vi "G Primitive to PLC Byte Stream.vi"(6 "Byte Length":i32, 8 "error in (no error)":errorcluster, 9 "PLC Type":T1, 10 "Value":variant, 11 "TwinCAT ADS in":refnum<class "TwinCAT ADS.lvclass">) -> (0 "error out":errorcluster, 2 "Byte Stream":u8[](array[numeric]), 3 "TwinCAT ADS out":refnum<class "TwinCAT ADS.lvclass">)   [LabVIEW 2018, in "TwinCAT ADS.lvclass"]
uses:
  TwinCAT ADS.lvclass
  Controls/PLC Type.ctl
  ebfc1059-5ad7-41af-9a32-6ba056cec1e2.vi
  6e01a951-886b-41b5-8cd1-fdd71fd1a533.vi
  09c7a0ef-3209-4624-b801-f77696e71225.vi
  97b8602c-6a72-408e-90bf-08a26de32539.vi
  0fd4fbf3-4a18-432c-8f70-6a5c8fef8454.vi
  afdb5a5e-237c-4be5-828e-15f510cf6cea.vi
  185a6e12-4d7d-4ad7-9936-0525adb2f85e.vi
  88229fb8-b58c-494b-bd2b-fea6e0d0ed1b.vi
  e57df404-389c-41d0-a67c-37c75754ab31.vi
  d0ee652c-9b86-46ed-9065-57d03aa8de3e.vi
  886bf0b9-f01c-4a44-b2e2-abccc7b97bfa.vi
  35f71df7-fc14-4c4d-983c-cf72c138dc9e.vi
  2d2bc992-a9ff-4dd8-b8fe-74c21cb85899.vi
  100e4a11-5e4a-45b7-be98-adc9eaebd48d.vi
  132946d9-68c7-4ade-a66d-dc369520c644.vi
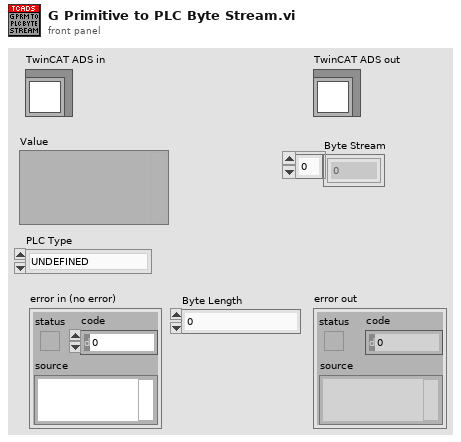
[diagram p1: front panel]
types:
  T1 = typedef "TwinCAT ADS.lvclass/PLC Type.ctl" = enum16{"UNDEFINED", "INT", "DINT", "REAL", "LREAL", "SINT", "BYTE", "UINT", "UDINT", "LINT", "ULINT", "STRING", "WSTRING", "BOOL", "TIME", "LTIME", "DATE", "DT", "TOD", "ARRAY", "JAGGED ARRAY", "STRUCT", "FUNCTION BLOCK", "UNION", "POINTER", "USER DEFINED"}
  T2 = typedef "LVDateTimeRec.ctl" = cluster{"fractional second":dbl, "second":i32, "minute":i32, "hour":i32, "day of month":i32, "month":i32, "year":i32, "day of week":i32, "day of year":i32, "DST":i32}
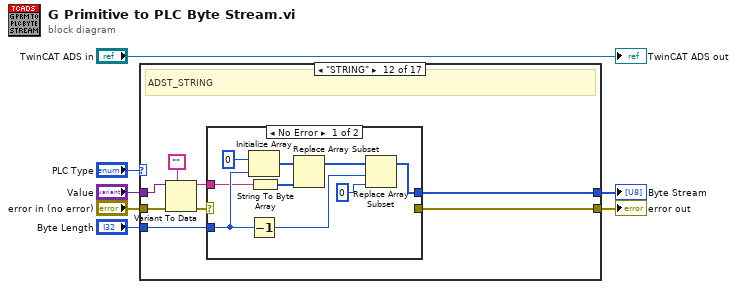
[diagram p0: block diagram]
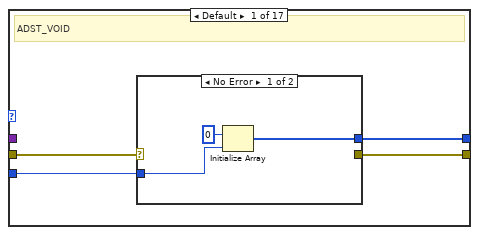
[diagram p2: hidden frame]
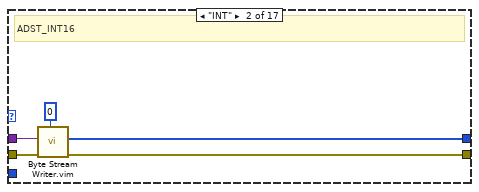
[diagram p4: hidden frame]
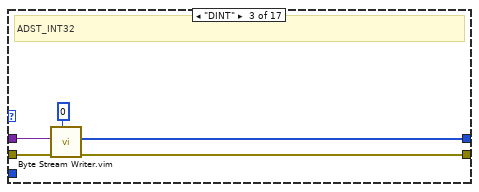
[diagram p5: hidden frame]
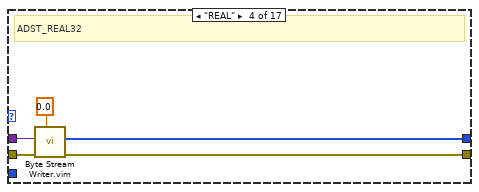
[diagram p6: hidden frame]
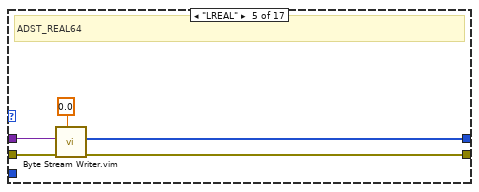
[diagram p7: hidden frame]
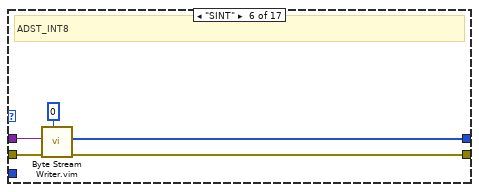
[diagram p8: hidden frame]
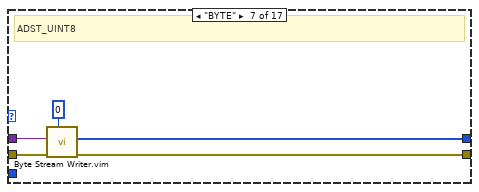
[diagram p9: hidden frame]
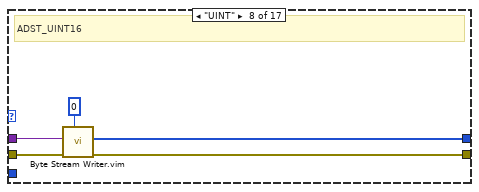
[diagram p10: hidden frame]
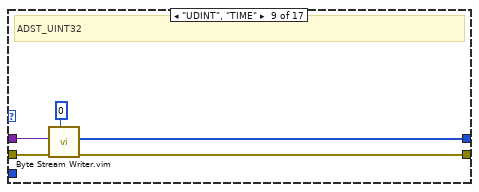
[diagram p11: hidden frame]
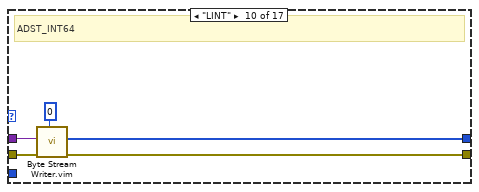
[diagram p12: hidden frame]
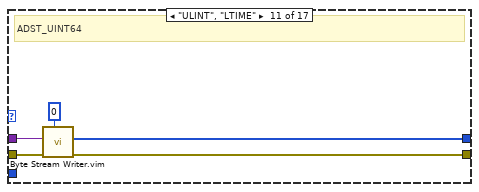
[diagram p13: hidden frame]
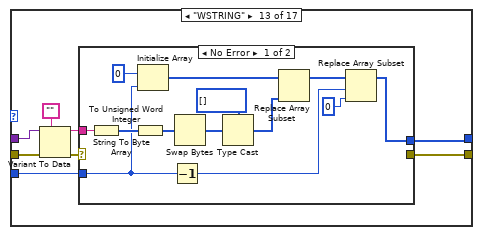
[diagram p15: hidden frame]
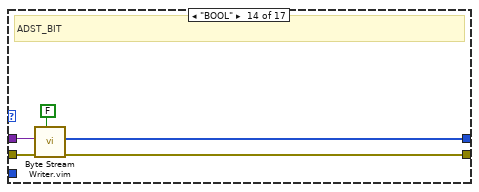
[diagram p17: hidden frame]
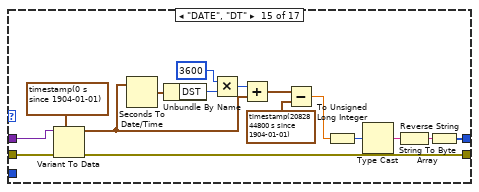
[diagram p18: hidden frame]
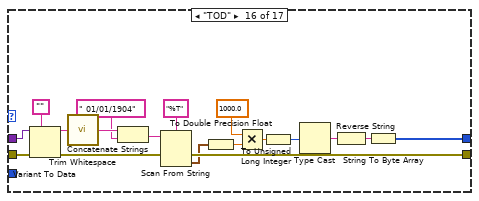
[diagram p19: hidden frame]
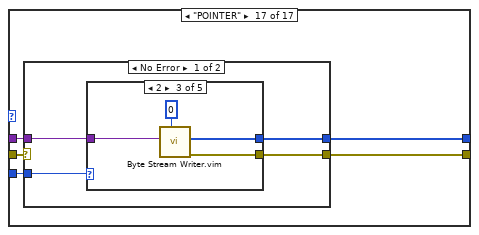
[diagram p20: hidden frame]
diagram:
  n1 = case shown="\"STRING\"" "PLC Type" {
    tunnel: "error in (no error)" -> [w9 w20 w25 w30 w34 w40 w45 w50 w55 w60 w65 w72 w89 w110 w126 w143 w146]
    tunnel: [w8 w17 w23 w27 w32 w37 w42 w47 w54 w57 w62 w67 w84 w107 w119 w144 w145] -> w6
    tunnel: "Value" -> [_ w19 w24 w29 w33 w39 w44 w49 w51 w59 w64 w71 w88 w109 w125 w141 w147]
    tunnel: [w10 w16 w21 w26 w31 w36 w41 w46 w53 w56 w61 w66 w91 w106 w111 w139 w148] -> w4
    tunnel: "Byte Length" -> [w11 _ _ _ _ _ _ _ _ _ _ w73 w90 _ _ _ w149]
    frame Default {
      # "ADST_VOID"
      n2 = case shown="No Error" w9 {
        selector: w9 -> [_ w15]
        tunnel: w11 -> [w13 _]
        tunnel: [w12 _] -> w10
        tunnel: [_ w15] -> w8
        frame No Error {
          n3 = Initialize Array(u8 0, w13) -> (w12:u8[])
        }
        frame Error {
        }
      }
    }
    frame "INT" {
      # "ADST_INT16"
      n4 = call "Byte Stream Writer.vim"("Type"=i16 0, "error in (no error)"=w20, "Value"=w19) -> ("error out"=w17:errorcluster, "Byte Stream"=w16:u8[])  [unwired: 7 in]
    }
    frame "DINT" {
      # "ADST_INT32"
      n5 = call "Byte Stream Writer.vim"("Type"=0, "error in (no error)"=w25, "Value"=w24) -> ("error out"=w23:errorcluster, "Byte Stream"=w21:u8[])  [unwired: 7 in]
    }
    frame "REAL" {
      # "ADST_REAL32"
      n6 = call "Byte Stream Writer.vim"("Type"=sgl 0.0, "error in (no error)"=w30, "Value"=w29) -> ("error out"=w27:errorcluster, "Byte Stream"=w26:u8[])  [unwired: 7 in]
    }
    frame "LREAL" {
      # "ADST_REAL64"
      n7 = call "Byte Stream Writer.vim"("Type"=0.0, "error in (no error)"=w34, "Value"=w33) -> ("error out"=w32:errorcluster, "Byte Stream"=w31:u8[])  [unwired: 7 in]
    }
    frame "SINT" {
      # "ADST_INT8"
      n8 = call "Byte Stream Writer.vim"("Type"=i8 0, "error in (no error)"=w40, "Value"=w39) -> ("error out"=w37:errorcluster, "Byte Stream"=w36:u8[])  [unwired: 7 in]
    }
    frame "BYTE" {
      # "ADST_UINT8"
      n9 = call "Byte Stream Writer.vim"("Type"=u8 0, "error in (no error)"=w45, "Value"=w44) -> ("error out"=w42:errorcluster, "Byte Stream"=w41:u8[])  [unwired: 7 in]
    }
    frame "UINT" {
      # "ADST_UINT16"
      n10 = call "Byte Stream Writer.vim"("Type"=u16 0, "error in (no error)"=w50, "Value"=w49) -> ("error out"=w47:errorcluster, "Byte Stream"=w46:u8[])  [unwired: 7 in]
    }
    frame "UDINT", "TIME" {
      # "ADST_UINT32"
      n11 = call "Byte Stream Writer.vim"("Type"=u32 0, "error in (no error)"=w55, "Value"=w51) -> ("error out"=w54:errorcluster, "Byte Stream"=w53:u8[])  [unwired: 7 in]
    }
    frame "LINT" {
      # "ADST_INT64"
      n12 = call "Byte Stream Writer.vim"("Type"=i64 0, "error in (no error)"=w60, "Value"=w59) -> ("error out"=w57:errorcluster, "Byte Stream"=w56:u8[])  [unwired: 7 in]
    }
    frame "ULINT", "LTIME" {
      # "ADST_UINT64"
      n13 = call "Byte Stream Writer.vim"("Type"=u64 0, "error in (no error)"=w65, "Value"=w64) -> ("error out"=w62:errorcluster, "Byte Stream"=w61:u8[])  [unwired: 7 in]
    }
    frame "STRING" {
      # "ADST_STRING"
      n14 = Variant To Data(error in=w72, type="", Variant=w71) -> (data=w69:string, error out=w68:errorcluster)
      n15 = case shown="No Error" w68 {
        selector: w68 -> [_ w83]
        tunnel: w73 -> [w79 _]
        tunnel: w69 -> [w78 _]
        tunnel: [_ w83] -> w67
        tunnel: [w74 _] -> w66
        frame No Error {
          n16 = Initialize Array(u8 0 ("element"), w79) -> (w77:u8[])
          n17 = Decrement(x=w79) -> (x-1=w81:i32)
          n18 = String To Byte Array(string=w78) -> (unsigned byte array=w76:u8[])
          n19 = Replace Array Subset(array=w77, new element=w76) -> (w75:u8[])  [unwired: 1 in]
          n20 = Replace Array Subset(array=w75, new element=u8 0 ("new element/subarray"), index=w81) -> (w74:u8[])
        }
        frame Error {
        }
      }
    }
    frame "WSTRING" {
      n21 = Variant To Data(error in=w89, type="", Variant=w88) -> (data=w86:string, error out=w85:errorcluster)
      n22 = case shown="No Error" w85 {
        selector: w85 -> [_ w105]
        tunnel: [w92 _] -> w91
        tunnel: w90 -> [w95 _]
        tunnel: w86 -> [w99 _]
        tunnel: [_ w105] -> w84
        frame No Error {
          n23 = String To Byte Array(string=w99) -> (unsigned byte array=w103:u8[])
          n24 = To Unsigned Word Integer(number=w103) -> (unsigned 16bit integer=w96:u16[])
          n25 = Initialize Array(u8 0, w95) -> (w101:u8[])
          n26 = Decrement(x=w95) -> (x-1=w94:i32)
          n27 = Swap Bytes(anything=w96) -> (byte swapped=w98:u16[])
          n28 = Type Cast(type=u8[] [] ("initialized array"), x=w98) -> (*(type *) &x=w100:u8[])
          n29 = Replace Array Subset(array=w101, new element=w100) -> (w97:u8[])  [unwired: 1 in]
          n30 = Replace Array Subset(array=w97, new element=u8 0 ("new element/subarray"), index=w94) -> (w92:u8[])
        }
        frame Error {
        }
      }
    }
    frame "BOOL" {
      # "ADST_BIT"
      n31 = call "Byte Stream Writer.vim"("Type"=FALSE, "error in (no error)"=w110, "Value"=w109) -> ("error out"=w107:errorcluster, "Byte Stream"=w106:u8[])  [unwired: 7 in]
    }
    frame "DATE", "DT" {
      n32 = Variant To Data(error in=w126, type=timestamp(0 s since 1904-01-01), Variant=w125) -> (data=w113:timestamp, error out=w119:errorcluster)
      n33 = Seconds To Date/Time(time stamp (now)=w113) -> (date time rec=w123:T2)  [unwired: 1 in]
      n34 = Unbundle By Name(w123) -> ("DST"=w121:i32)
      n35 = Multiply(x=3600, y=w121) -> (x*y=w122:i32)
      n36 = Add(x=w122, y=w113) -> (x+y=w124:timestamp)
      n37 = Subtract(x=w124, y=timestamp(2082844800 s since 1904-01-01) ("time stamp")) -> (x-y=w114:dbl)
      n38 = To Unsigned Long Integer(number=w114) -> (unsigned 32bit integer=w118:u32)
      n39 = Type Cast(x=w118) -> (*(type *) &x=w116:string)  [unwired: 1 in]
      n40 = Reverse String(1:w116) -> (0:w117:string)
      n41 = String To Byte Array(string=w117) -> (unsigned byte array=w111:u8[])
    }
    frame "TOD" {
      n42 = Variant To Data(error in=w143, type="", Variant=w141) -> (data=w138:string, error out=w142:errorcluster)
      n43 = call <vilib>:"Trim Whitespace.vi"("string"=w138) -> ("trimmed string"=w135:string)  [unwired: 1 in]
      n44 = Concatenate Strings(w135, " 01/01/1904") -> (w134:string)
      n45 = Scan From String(format string="%T", input string=w134, error in=w142) -> (error out=w144:errorcluster, output 1=w132:timestamp)  [unwired: 2 in, 2 out]
      n46 = To Double Precision Float(number=w132) -> (double precision float=w129:dbl)
      n47 = Multiply(x=1000.0 ("y"), y=w129) -> (x*y=w136:dbl)
      n48 = To Unsigned Long Integer(number=w136) -> (unsigned 32bit integer=w127:u32)
      n49 = Type Cast(x=w127) -> (*(type *) &x=w131:string)  [unwired: 1 in]
      n50 = Reverse String(1:w131) -> (0:w130:string)
      n51 = String To Byte Array(string=w130) -> (unsigned byte array=w139:u8[])
    }
    frame "POINTER" {
      n52 = case shown="No Error" w146 {
        selector: w146 -> [_ w173]
        tunnel: w149 -> [w153 _]
        tunnel: [w152 _] -> w148
        tunnel: w147 -> [w151 _]
        tunnel: [w150 w173] -> w145
        frame No Error {
          n53 = case shown="2" w153 {
            selector: w153 -> [w156 _ _ _ _]
            tunnel: [w154 w158 w162 w166 w170] -> w152
            tunnel: w151 -> [_ w159 w163 w167 w171]
            tunnel: [_ w157 w161 w165 w169] -> w150
            frame Default {
              n54 = Initialize Array(u8 0, w156) -> (w154:u8[])
            }
            frame 1 {
              n55 = call "Byte Stream Writer.vim"("Type"=u8 0, "Value"=w159) -> ("error out"=w157:errorcluster, "Byte Stream"=w158:u8[])  [unwired: 8 in]
            }
            frame 2 {
              n56 = call "Byte Stream Writer.vim"("Type"=u16 0, "Value"=w163) -> ("error out"=w161:errorcluster, "Byte Stream"=w162:u8[])  [unwired: 8 in]
            }
            frame 4 {
              n57 = call "Byte Stream Writer.vim"("Type"=u32 0, "Value"=w167) -> ("error out"=w165:errorcluster, "Byte Stream"=w166:u8[])  [unwired: 8 in]
            }
            frame 8 {
              n58 = call "Byte Stream Writer.vim"("Type"=u64 0, "Value"=w171) -> ("error out"=w169:errorcluster, "Byte Stream"=w170:u8[])  [unwired: 8 in]
            }
          }
        }
        frame Error {
        }
      }
    }
  }
  "error out" <- w6
  "Byte Stream" <- w4
  "TwinCAT ADS out" <- "TwinCAT ADS in"
